vi "emi_Set Debug status.vi"(1 "Debug Disp":bool, 2 "Debug Log":bool, 3 "Debug Aditional":bool, 9 "error in (no error)":errorcluster) -> (10 "error out":errorcluster)   [LabVIEW 2011]
doc: "Checks wheter the application id closeing,"
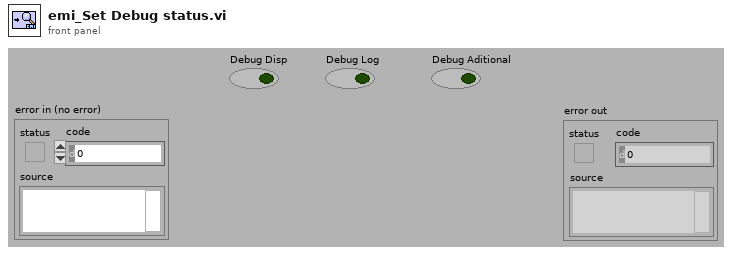
[diagram p1: front panel]
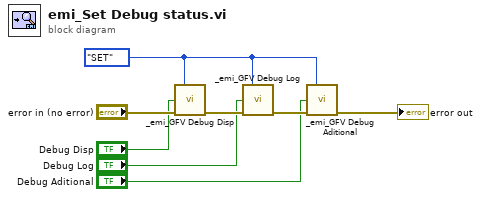
[diagram p0: block diagram]
diagram:
  w3 = enum16{"GET", "SET"}."SET" ("Action(GET)")
  n1 = call "_emi_GFV Debug Disp.vi"("Action(GET)"=w3, "Debug Disp"="Debug Disp", "error in (no error)"="error in (no error)") -> ("error out"=w7:errorcluster)  [unwired: 11 in, 1 out]
  n2 = call "_emi_GFV Debug Log.vi"("Action(GET)"=w3, "Debug Log"="Debug Log", "error in (no error)"=w7) -> ("error out"=w6:errorcluster)  [unwired: 11 in, 1 out]
  n3 = call "_emi_GFV Debug Aditional.vi"("Action(GET)"=w3, "Debug Aditional"="Debug Aditional", "error in (no error)"=w6) -> ("error out"=→"error out":errorcluster)  [unwired: 11 in, 1 out]
